vi "KeepGoingUntilPosReached4Axes.vi"(7 "Variables d'Axes":T1={"OrdreBloc"="ni.var.psp://localhost/OPC/OPC1/esbimETH_1/module1/2AXBOC/E0_Ordre/Axe2_OrdreBloc", "Ordre UC"="ni.var.psp://localhost/OPC/OPC1/esbimETH_1/module1/2AXBOC/E0_Ordre/Axe2_OrdreUC", "CoteAAtteindre"="ni.var.psp://localhost/OPC/OPC1/esbimETH_1/module1/2AXBOC/E2_Position2/CoteAAtteindre", "Vitesse"="ni.var.psp://localhost/OPC/OPC1/esbimETH_1/module1/2AXBOC/E2_Position2/Vitesse", "Position codeur en pas"="ni.var.psp://localhost/OPC/OPC1/esbimETH_1/module1/2AXBOC/L4_PositionPas/Axe2_PositionCodeurEnPas", "Position Théorique"="ni.var.psp://localhost/OPC/OPC1/esbimETH_1/module1/2AXBOC/L0_Position/Axe2_PositionTheorique", "Message"="ni.var.psp://localhost/OPC/OPC1/esbimETH_1/module1/2AXBOC/L0_Position/Axe2_Messages", "Ecrire"="ni.var.psp://localhost/OPC/OPC1/esbimETH_1/module1/2AXBOC/ecrire", "Zone à écrire"="ni.var.psp://localhost/OPC/OPC1/esbimETH_1/module1/2AXBOC/zones_a_ecrire", "Numéro paramètre"="ni.var.psp://localhost/OPC/OPC1/esbimETH_1/module1/2AXBOC/E3_Parametres/NumeroParametre", "Ordre"="ni.var.psp://localhost/OPC/OPC1/esbimETH_1/module1/2AXBOC/E3_Parametres/Ordre", "Valeur"="ni.var.psp://localhost/OPC/OPC1/esbimETH_1/module1/2AXBOC/E3_Parametres/Valeur", "Valeur Lecture"="ni.var.psp://localhost/OPC/OPC1/esbimETH_1/module1/2AXBOC/L2_Parametres/Valeur", "Numéro paramètre Lecture"="ni.var.psp://localhost/OPC/OPC1/esbimETH_1/module1/2AXBOC/L2_Parametres/Numero", "Acquittement Lecture Ecriture"="ni.var.psp://localhost/OPC/OPC1/esbimETH_1/module1/2AXBOC/L2_Parametres/AcquitementLectureEcriture", "Zone à Ecrire Pour Axe "=0, "Acquittement Ordre UC"=""}, 8 "error in (no error)":errorcluster caption="entrée d'erreur (pas d'erreur)", 9 "Cote à atteindre":i32, 10 "Axe?":enum16{"Axe1", "Axe2", "Axe3", "Axe4"}(ring)) -> (0 "error out":errorcluster caption="sortie d'erreur", 1 "Nombre d'essais":i32)   [LabVIEW 2013]
uses:
  Controls/AdressesVariablesPartagees.ctl
  Commandes/Type de Mouvement PilMOT.ctl
panel:
  out "Axe1_Messages":u16
  out "Message Axe":string
  in  "Axe4_PositionCodeurEnPas":i32
  in  "Axe3_PositionCodeurEnPas":i32
  in  "Axe2_PositionCodeurEnPas":i32
  in  "Axe1_PositionCodeurEnPas":i32
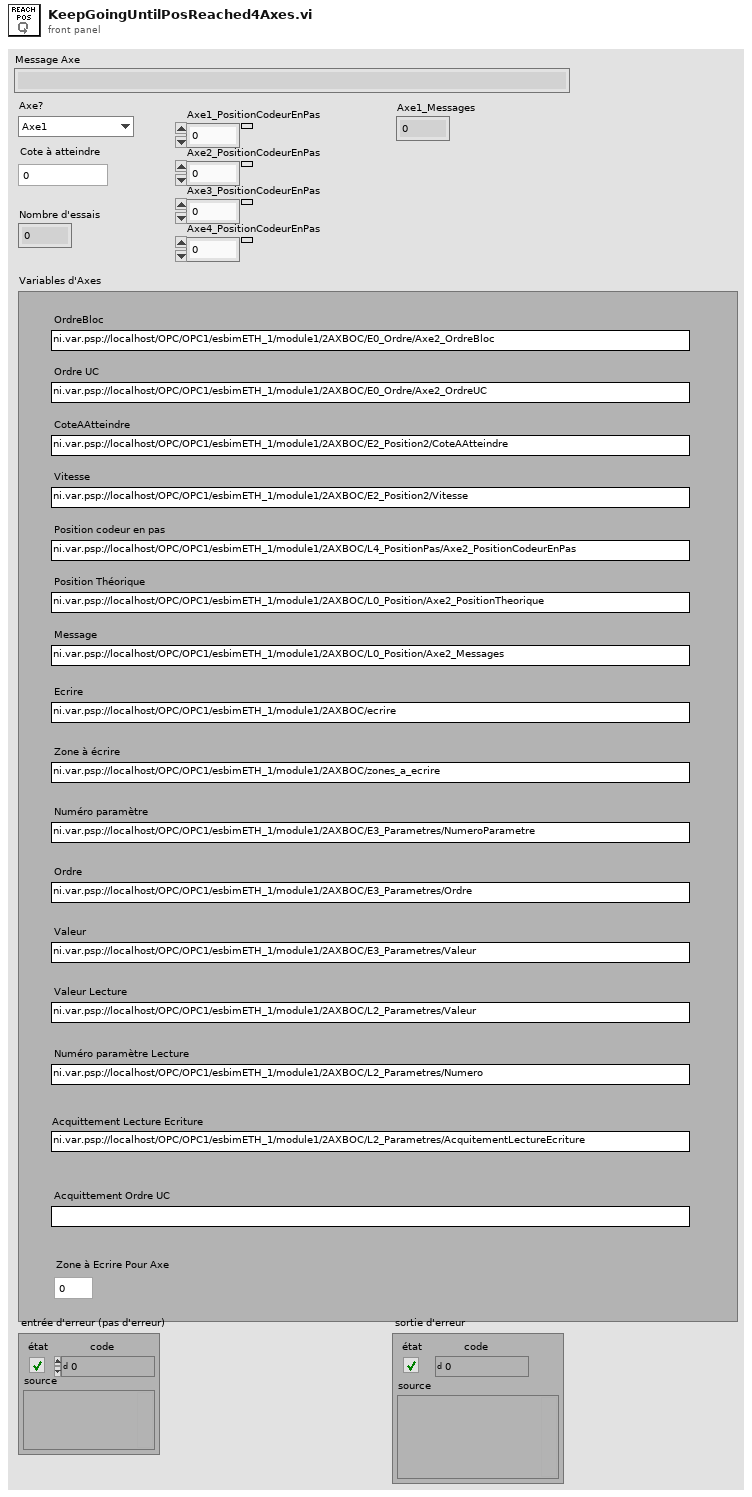
[diagram p1: front panel]
types:
  T1 = typedef "AdressesVariablesPartagees.ctl" = cluster{"OrdreBloc":string, "Ordre UC":string, "CoteAAtteindre":string, "Vitesse":string, "Position codeur en pas":string, "Position Théorique":string, "Message":string, "Ecrire":string, "Zone à écrire":string, "Numéro paramètre":string, "Ordre":string, "Valeur":string, "Valeur Lecture":string, "Numéro paramètre Lecture":string, "Acquittement Lecture Ecriture":string, "Zone à Ecrire Pour Axe ":u16, "Acquittement Ordre UC":string}
  T2 = typedef "Type de Mouvement PilMOT.ctl" = u16
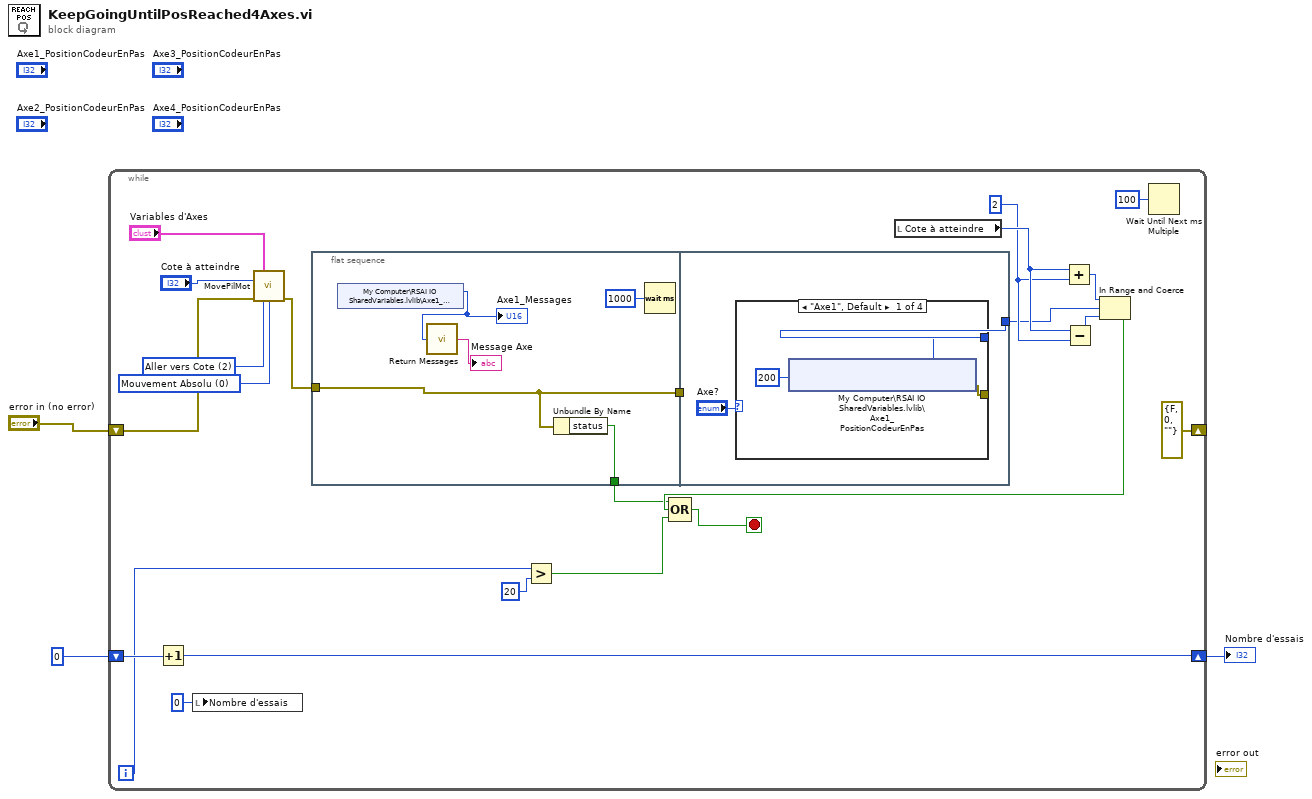
[diagram p0: block diagram]
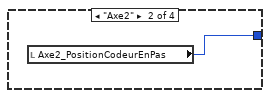
[diagram p2: hidden frame]
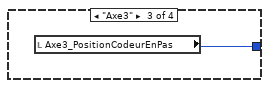
[diagram p3: hidden frame]
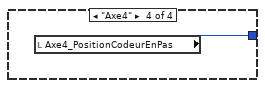
[diagram p4: hidden frame]
diagram:
  n1 = while {
    shift-right: [errorcluster {"status"=FALSE, "code"=0, "source"=""} ("error in (no error)")] -> _
    shift-left: "error in (no error)" -> [w25]
    shift-right: [w17] -> w1
    shift-left: 0 -> [w18]
    i -> [w8]
    stop <- w9 stop-if-true
    w12 = 2 ("Cote à atteindre")
    w23 = u16 0 items=["Mouvement Relatif"=1, "Mouvement Absolu"=0] ("Mouvement Absolu/Relatif")
    w24 = T2 2 items=["Mouvement Simple"=1, "Aller vers Cote"=2, "Va vers position de référence"=3] ("Type de mouvement")
    n2 = Increment(x=w18) -> (x+1=w17:i32)
    n3 = local write "Nombre d'essais"(0 ("Nombre d'essais")) -> ()
    n4 = call "MovePilMot.vi"("Variables d'Axes"="Variables d'Axes", "Cote à atteindre"="Cote à atteindre", "error in (no error)"=w25, "Type de mouvement"=w24, "Mouvement Absolu/Relatif"=w23) -> ("error out"=w21:errorcluster)  [unwired: 10 in]
    n5 = flat-sequence {
      tunnel: w21 -> [w28]
      tunnel: [w28] -> w6
      tunnel: [w27] -> w4
      tunnel: w6 -> [_]
      tunnel: [w32] -> w5
      frame #0 {
        n6 = shared-variable "My Computer\\RSAI IO SharedVariables.lvlib\\Axe1_Messages"() -> (w31:u16)  [unwired: 1 in, 1 out]
        "Axe1_Messages" <- w31
        n7 = call "Return Messages.vi"("Nombre à convertir"=w31) -> ("Message Axe"=→"Message Axe":string)
        n8 = Unbundle By Name(w28) -> ("status"=w27:bool)
        n9 = Wait (ms)(milliseconds to wait=u32 1000 ("attente (ms)")) -> ()  [unwired: 1 out]
      }
      frame #1 {
        n10 = case shown="\"Axe1\", Default" "Axe?" {
          tunnel: [w35 w37 w38 w39] -> w32
          tunnel: [w36 _ _ _] -> _
          frame "Axe1", Default {
            n11 = shared-variable "My Computer\\RSAI IO SharedVariables.lvlib\\Axe1_PositionCodeurEnPas"(200 ("ms timeout (0)")) -> (w35:i32, error out=w36:errorcluster)  [unwired: 1 in, 1 out]
          }
          frame "Axe2" {
            n12 = local read "Axe2_PositionCodeurEnPas"() -> (w37:i32)
          }
          frame "Axe3" {
            n13 = local read "Axe3_PositionCodeurEnPas"() -> (w38:i32)
          }
          frame "Axe4" {
            n14 = local read "Axe4_PositionCodeurEnPas"() -> (w39:i32)
          }
        }
      }
    }
    n15 = Greater?(x=w8, y=20 ("x")) -> (0:w20:bool)
    n16 = local read "Cote à atteindre"() -> (w13:i32)
    n17 = Add(x=w13, y=w12) -> (x+y=w15:i32)
    n18 = Subtract(x=w13, y=w12) -> (x-y=w14:i32)
    n19 = In Range and Coerce(upper limit=w15, x=w5, lower limit=w14) -> (In Range?=w11:bool)  [unwired: 1 out]
    n20 = Compound Arithmetic op=OR(w4, w11, w20) -> (w9:bool)
    n21 = Wait Until Next ms Multiple(millisecond multiple=u32 100 ("milliseconds to wait")) -> ()  [unwired: 1 out]
  }
  "Nombre d'essais" <- w1
